vi "digital galvo ADC.vi"(9 "zero point":i32=32768, 11 "Analog waveform":dbl[](array[numeric])) -> (3 "Digital waveform":bool[](array[boolean]))   [LabVIEW 2015]
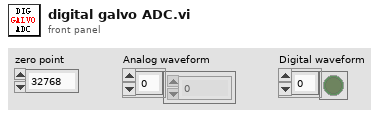
[diagram p1: front panel]
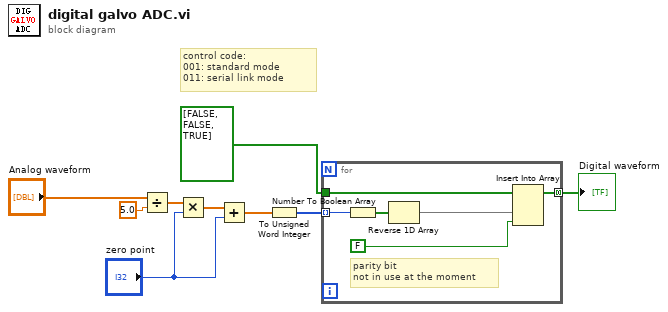
[diagram p0: block diagram]
diagram:
  # "control code:\n001: standard mode\n011: serial link mode"
  n1 = Divide(x="Analog waveform", y=5.0) -> (x/y=w7:dbl[])
  n2 = Multiply(x=w7, y="zero point") -> (x*y=w6:dbl[])
  n3 = Add(x=w6, y="zero point") -> (x+y=w5:dbl[])
  n4 = To Unsigned Word Integer(number=w5) -> (unsigned 16bit integer=w4:u16[])
  n5 = for {
    tunnel: w4 -> [w15] mode=indexing
    tunnel: bool[] [FALSE, FALSE, TRUE] ("Array") -> [w12]
    tunnel: [w10] -> w2 mode=concatenating
    # "parity bit\nnot in use at the moment"
    n6 = Number To Boolean Array(number=w15) -> (Boolean array=w14:bool[])
    n7 = Reverse 1D Array(array=w14) -> (reversed array=w13:bool[])
    n8 = Insert Into Array(array=w12, new element #1=w13, new element #2=FALSE ("new element/subarray")) -> (w10:bool[])  [unwired: 1 in]
  }
  "Digital waveform" <- w2
